vi "writeSketch.vi"(9 "Code":string, 10 "File name":string, 11 "path to ino folder":path) -> (2 "Sketch.ino":string, 3 "path to ino file":path)   [LabVIEW 2020]
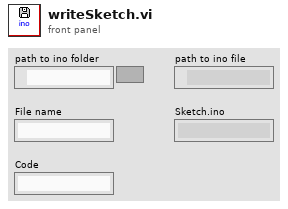
[diagram p1: front panel]
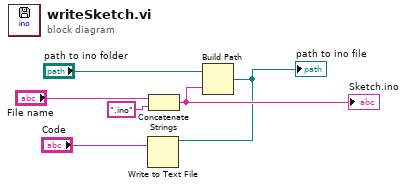
[diagram p0: block diagram]
diagram:
  n1 = Concatenate Strings("File name", ".ino" ("string")) -> (w4:string)
  "Sketch.ino" <- w4
  n2 = Build Path(base path="path to ino folder", name or relative path=w4) -> (appended path=w1:path)
  "path to ino file" <- w1
  n3 = Write to Text File(file (use dialog)=w1, text="Code") -> ()  [unwired: 2 in, 3 out]
